vi "Impulse Analyser Top Stack.vi"(2 "State stack IN":T1[](array[typedef])) -> (0 "State stack OUT":T1[](array[typedef]), 1 "State":T1=enum."Panel Monitoring")   [LabVIEW 2016]
uses:
  Impulse Analyser state.ctl
panel:
  # "Top Stack\nVER 1.0 AAM 10th April 2002\n\nThis VI removes the top element of the state stack \nand returns the remaining elements in the stack"
  # "Copyright Americo A. Migliaccio (c) 2002 All Rights Reserved by Author"
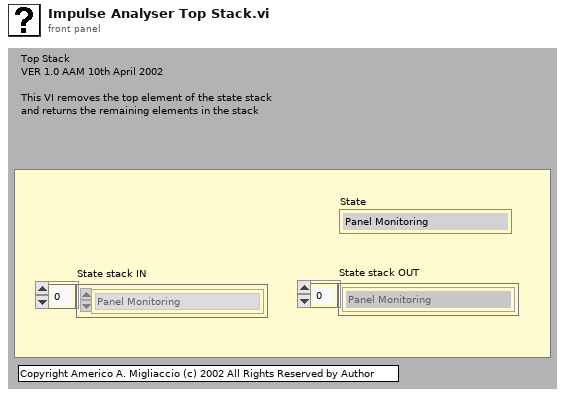
[diagram p1: front panel]
types:
  T1 = typedef "Impulse Analyser state.ctl" = enum16{"--- System ---", "Panel Monitoring", "Initialize", "Initialise GUI", "Quit", "--- Import ---", "Desaccade Time Data", "Desaccade Time Data Background", "Paint Delete", "Load Batch Log File", "Update Batch List", "Delete Batch List", "Delete Temporary LVS", "Save Temporary LVS", "Check for Batch LVS", "Process 3D Chinchilla", "Find default parameter", "Mars3D old", "Chair", "EyeSeeCam", "Open last session", "Save RAW", "Auto Impulse Parameter", "Save Image", "Wireless", "Process Coils Data", "Process JHOC Data", "Process Animal Data", "Australian Data", "ASCII", "Mars 3D", "Mars 3D Training", "Position Mean Plugin", "plot generator plugin", "Human VOG system", "Optotrak", "spline", "COR", "galvanic", "Generate New Time Plot", "Make off and gains permanent", "Generate New Impulse Plot", "Generate New Impulse Plot (No Scaling)", "Defer Impulse Plot", "Fill Impulse Plot Data", "Scale Impulse Plot", "Un-Defer Impulse Plot", "Snap Impulse Cursor", "Extract Saccades", "Impulse Analyser", "NTA", "Acceleration", "Saccade Velocity", "Horizontal Align", "Vertical Align", "Delete Impulse", "Cut Before", "Cut After", "Filter Data", "Mean and STD", "Generate Report", "Phase Plots", "Gain and Phase", "Example Plugin", "Time Constant Plugin", "Export Data", "Export Time Series Data", "Append Data", "Save Data", "Load Data", "Cut in Range", "Keep in range", "Advanced Cut"}
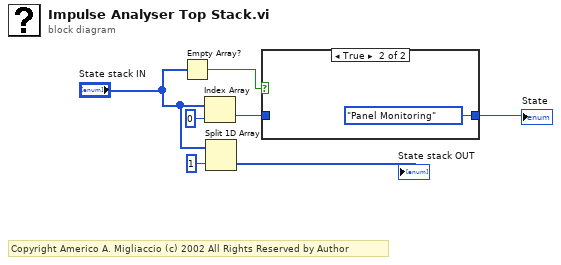
[diagram p0: block diagram]
diagram:
  # "Copyright Americo A. Migliaccio (c) 2002 All Rights Reserved by Author"
  n1 = Empty Array?(array="State stack IN") -> (empty?=w2:bool)
  n2 = Index Array(array="State stack IN", index=0) -> (element=w5:T1)
  n3 = Split 1D Array(array="State stack IN", index=1) -> (second subarray=→"State stack OUT":T1[])  [unwired: 1 out]
  n4 = case shown="True" w2 {
    tunnel: w5 -> [w8 _]
    tunnel: [w8 Impulse_Analyser_state."Panel Monitoring" ("State")] -> w1
    frame False {
    }
    frame True {
    }
  }
  "State" <- w1
